vi "Emballage_BDD_Select_portcom.vi"(8 "entrée d'erreur (pas d'erreur)":errorcluster, 9 "Famille":u16, 10 "Familles":string[](array[string])) -> (0 "sortie d'erreur":errorcluster, 3 "Refnum VISA en sortie":refnum<visa-resource-name>)   [LabVIEW 2020]
uses:
  Modules/FS/60_FS_Controles/60_FS_SetGet.ctl
  <vilib>/drjdpowell/SQLite Library/SQL Connection/Open (path).vi
  <vilib>/drjdpowell/SQLite Library/SQL Connection/Open (string).vi
  <vilib>/AdvancedString/Path To Command Line String.vi
  <vilib>/drjdpowell/SQLite Library/SQL Connection/Connection.lvclass
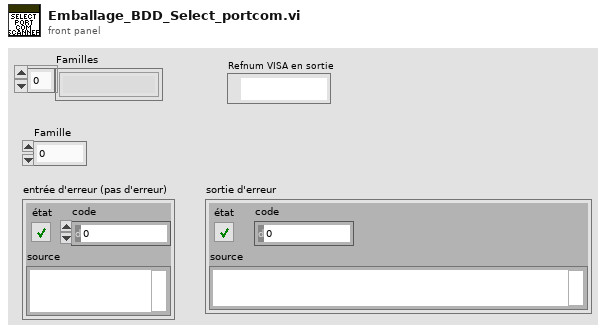
[diagram p1: front panel]
types:
  T1 = typedef "60_FS_SetGet.ctl" = enum16{"set", "get"}
  T2 = typedef "60_FS_CLT_Chemins.ctl" = cluster{"Racine_local":path, "Racine_reseau":path, "Racine_Support_Application":path, "Fichier_Journalisation":path, "Connexion_BDD_VSX":path, "Connexion_BDD_PLZ":path}
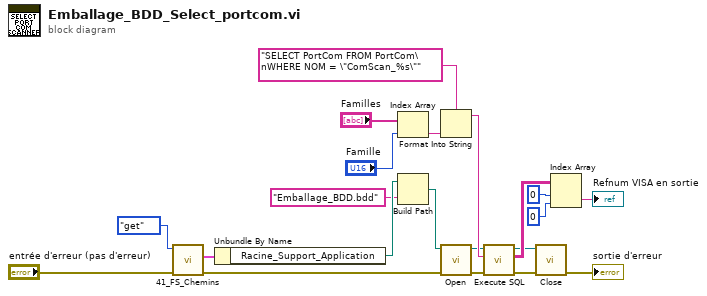
[diagram p0: block diagram]
diagram:
  n1 = call "41_FS_Chemins.vi"("error in (no error)"="entrée d'erreur (pas d'erreur)", "SetGet"=60_FS_SetGet."get") -> ("error out"=w13:errorcluster, "CLT_Chemins_out"=w15:T2)  [unwired: 8 in]
  n2 = Unbundle By Name(w15) -> ("Racine_Support_Application"=w14:path)
  n3 = Index Array(array="Familles", index="Famille") -> (element=w1:string)
  n4 = Build Path(base path=w14, name or relative path="Emballage_BDD.bdd" ("nom ou chemin relatif")) -> (appended path=w10:path)
  n5 = Format Into String(format string="SELECT PortCom FROM PortCom\nWHERE NOM = \"ComScan_%s\"" ("SQL"), w1) -> (resulting string=w17:string)  [unwired: 2 in, 1 out]
  n6 = call-poly <vilib>:"Open.vi"("error in (no error)"=w13, "db file"=w10) -> ("error out"=w12:errorcluster, "SQLite Connection"=w11:refnum<class "Connection.lvclass">)  [unwired: 8 in]
  n7 = call <vilib>:"Execute SQL.vi"("error in (no error)"=w12, "SQL"=w17, "SQLite Connection in"=w11) -> ("error out"=w4:errorcluster, "Result Set"=w8:string[][], "SQLite Connection"=w5:refnum<class "Connection.lvclass">)  [unwired: 5 in, 1 out]
  n8 = call-dynamic "Close.vi"("error in (no error)"=w4, "SQLite Connection in"=w5) -> ("error out"=→"sortie d'erreur":errorcluster)  [unwired: 9 in]
  n9 = Index Array(array=w8, index (row)=0 ("indice (ligne)"), index (col)=0 ("indice désactivé (col)")) -> (element=→"Refnum VISA en sortie":string)
